vi "Main.vi"() -> ()   [LabVIEW 2021]
uses:
  <vilib>/myRIO/Common/Instrument Driver Framework/myRIO v1.0/Encoder/typedefs/Encoder Signal Mode.ctl
  <vilib>/Platform/TimedLoop/XDataNode/timing_clust.ctl
  <vilib>/Platform/TimedLoop/XDataNode/nitl_modes.ctl
  <vilib>/Platform/TimedLoop/XDataNode/wakeup.ctl
  <vilib>/myRIO/Common/Instrument Driver Framework/myRIO v1.0/UART/vis/myRIO v1.0 Close UART.vi
  <vilib>/Utility/error.llb/Error Cluster From Error Code.vi
  <vilib>/myRIO/Common/Instrument Driver Framework/myRIO v1.0/Encoder/vis/myRIO v1.0 Read Encoder.vi
  <vilib>/myRIO/Common/Instrument Driver Framework/myRIO v1.0/DIO/vis/myRIO v1.0 Read DIO.vi
  <vilib>/myRIO/Common/Instrument Driver Framework/myRIO v1.0/PWM/vis/myRIO v1.0 Write PWM.vi
  <vilib>/myRIO/Common/Instrument Driver Framework/Utilities/vis/FPGA Ref Manager.vi
  <vilib>/myRIO/Common/Instrument Driver Framework/myRIO v1.0/myRIO v1.0 Reset FPGA.vi
  <vilib>/myRIO/Common/Instrument Driver Framework/myRIO v1.0/IRQ/vis/myRIO v1.0 IRQ Info FGV.vi
  <vilib>/myRIO/Common/Instrument Driver Framework/myRIO v1.0/IRQ/vis/myRIO v1.0 Timer IRQ Info FGV.vi
  <vilib>/myRIO/Common/Instrument Driver Framework/myRIO v1.0/IRQ/vis/myRIO v1.0 ISR Agent.vi
  <vilib>/myRIO/Instrument Drivers/Utilities/vis/Reset Index.vi
  <vilib>/myRIO/Common/Instrument Driver Framework/myRIO v1.0/Resource Manager/vis/myRIO v1.0 Block Write Resource Manager.vi
  <vilib>/Platform/TimedLoop/XDataNode/XDataNode.xnode
  <vilib>/myRIO/Instrument Drivers/Onboard IO/Encoder/Encoder.lvlib
  <vilib>/myRIO/Instrument Drivers/Onboard IO/PWM/PWM.lvlib
  <vilib>/myRIO/Instrument Drivers/Utilities/Utilities.lvlib
  <vilib>/Platform/TimedLoop/XDataNode/XDNodeRunTimeDep.lvlib
  <vilib>/myRIO/Instrument Drivers/Onboard IO/DIO/DIO.lvlib
panel:
  in  "Limit Switch":bool
  out "Saved Measurement":dbl
  in  "stop":bool
  in  "Measure":bool
  in  "X":dbl(slide) scale=0.0..50.0
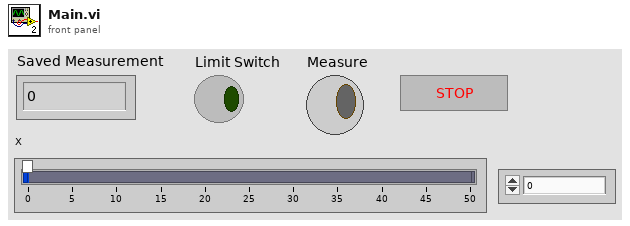
[diagram p1: front panel]
types:
  T1 = typedef "XDNodeRunTimeDep.lvlib/timing_clust.ctl" = cluster{"Expected End [f-1]":u64, "Actual End [f-1]":u64, "Finished Late? [f-1]":bool, "Expected End [i-1]":u64, "Actual End [i-1]":u64, "Finished Late? [i-1]":bool, "Expected Start [i]":u64, "Actual Start [i]":u64, "Expected Start [f]":u64, "Actual Start [f]":u64, "Source Name":string, "Structure Name":string, "Period":i64, "Deadline":i64, "Offset":i64, "Start":i64, "Priority":i32, "Timeout":i32, "Mode":T2, "Wakeup Reason":T3, "Error":errorcluster, "Source Type":string, "Secondary Source Type":string, "Global End Time":u64, "Global Start Time":u64, "Frame Duration":u64, "Iteration Duration":u64, "Assigned CPU":i32, "I/O Scan Engine Mode":u32}
  T2 = typedef "XDNodeRunTimeDep.lvlib/nitl_modes.ctl" = enum32{"No Change", "Process missed periods, maintain original phase", "Discard missed periods, maintain original phase", "Process missed periods, ignore original phase", "Discard missed periods, ignore original phase"}
  T3 = typedef "XDNodeRunTimeDep.lvlib/wakeup.ctl" = enum32{"Normal", "Aborted", "Asynchronous wakeup", "Timing source error", "Timed loop error", "Timeout"}
  T4 = enum8{"Enabled", "Disabled", "Disabled and Grayed Out"}
  T5 = typedef "Encoder Signal Mode.ctl" = enum16{"Quadrature phase signal", "Step and direction signal"}
  T6 = typedef "PWM.lvlib/PWM Reference.ctl" = cluster{"myRIO Reference":T7, "PWM Channels Enum":T11, "PWM Configuration":T12}
  T7 = typedef "myRIO Generic Hardware Reference.ctl" = cluster{"myRIO Model":T8, "myRIO Hardware Reference":T9}
  T8 = typedef "Hardware Version Enum.ctl" = enum16{"Unknown", "myRIO-1900", "myRIO-1950", "roboRIO", "NI ELVIS RIO CM", "ELVIS III"}
  T9 = typedef "myRIO v1.0 Reference.ctl" = cluster{"Generic FPGA Reference":T10, "Allow multiple opens":bool}
  T10 = typedef "Generic FPGA Reference.ctl" = refnum<k20>
  T11 = typedef "PWM Channels Enum.ctl" = enum16{"Not Connected", "C/PWM0", "C/PWM1", "A/PWM0", "A/PWM1", "A/PWM2", "A/PWM3", "A/PWM4", "A/PWM5", "A/PWM6", "A/PWM7", "A/PWM8", "A/PWM9", "A/PWM10", "A/PWM11", "A/PWM12", "A/PWM13", "A/PWM14", "A/PWM15", "A/PWM16", "A/PWM17", "A/PWM18", "A/PWM19", "B/PWM0", "B/PWM1", "B/PWM2", "B/PWM3", "B/PWM4", "B/PWM5", "B/PWM6", "B/PWM7", "B/PWM8", "B/PWM9", "B/PWM10", "B/PWM11", "B/PWM12", "B/PWM13", "B/PWM14", "B/PWM15", "B/PWM16", "B/PWM17", "B/PWM18", "B/PWM19", "PWM/PWM0", "PWM/PWM1", "PWM/PWM2", "PWM/PWM3", "PWM/PWM4", "PWM/PWM5", "PWM/PWM6", "PWM/PWM7", "PWM/PWM8", "PWM/PWM9"}
  T12 = typedef "PWM.lvlib/PWM Configuration.ctl" = cluster{"Frequency":dbl, "Duty Cycle":dbl}
  T13 = typedef "Encoder.lvlib/Encoder Reference.ctl" = cluster{"myRIO Reference":T7, "Encoder Channels Enum":T14}
  T14 = typedef "Encoder Channels Enum.ctl" = enum16{"Not Connected", "C/ENC0", "C/ENC1", "A/ENC", "A/ENC0", "A/ENC1", "A/ENC2", "A/ENC3", "A/ENC4", "A/ENC5", "A/ENC6", "A/ENC7", "A/ENC8", "A/ENC9", "B/ENC", "B/ENC0", "B/ENC1", "B/ENC2", "B/ENC3", "B/ENC4", "B/ENC5", "B/ENC6", "B/ENC7", "B/ENC8", "B/ENC9", "DIO/ENC0", "DIO/ENC1", "DIO/ENC2", "DIO/ENC3", "DIO/ENC4"}
  T15 = typedef "DIO.lvlib/DIO Reference.ctl" = cluster{"myRIO Reference":T7, "DIO Channels List":T16}
  T16 = typedef "DIO Channels List.ctl" = T17[]
  T17 = typedef "DIO Channels Enum.ctl" = enum16{"Not Connected", "C/DIO0", "C/DIO1", "C/DIO2", "C/DIO3", "C/DIO4", "C/DIO5", "C/DIO6", "C/DIO7", "A/DIO0", "A/DIO1", "A/DIO2", "A/DIO3", "A/DIO4", "A/DIO5", "A/DIO6", "A/DIO7", "A/DIO8", "A/DIO9", "A/DIO10", "A/DIO11", "A/DIO12", "A/DIO13", "A/DIO14", "A/DIO15", "A/DIO16", "A/DIO17", "A/DIO18", "A/DIO19", "B/DIO0", "B/DIO1", "B/DIO2", "B/DIO3", "B/DIO4", "B/DIO5", "B/DIO6", "B/DIO7", "B/DIO8", "B/DIO9", "B/DIO10", "B/DIO11", "B/DIO12", "B/DIO13", "B/DIO14", "B/DIO15", "B/DIO16", "B/DIO17", "B/DIO18", "B/DIO19", "LED0", "LED1", "LED2", "LED3", "Button0", "DIO/DIO0", "DIO/DIO1", "DIO/DIO2", "DIO/DIO3", "DIO/DIO4", "DIO/DIO5", "DIO/DIO6", "DIO/DIO7", "DIO/DIO8", "DIO/DIO9", "SPI/CS0", "SPI/CS1", "SPI/CS2", "SPI/CS3", "LED RADIO (Green)", "LED RADIO (Red)", "LED COMM (Green)", "LED COMM (Red)", "LED MODE (Green)", "LED MODE (Red)"}
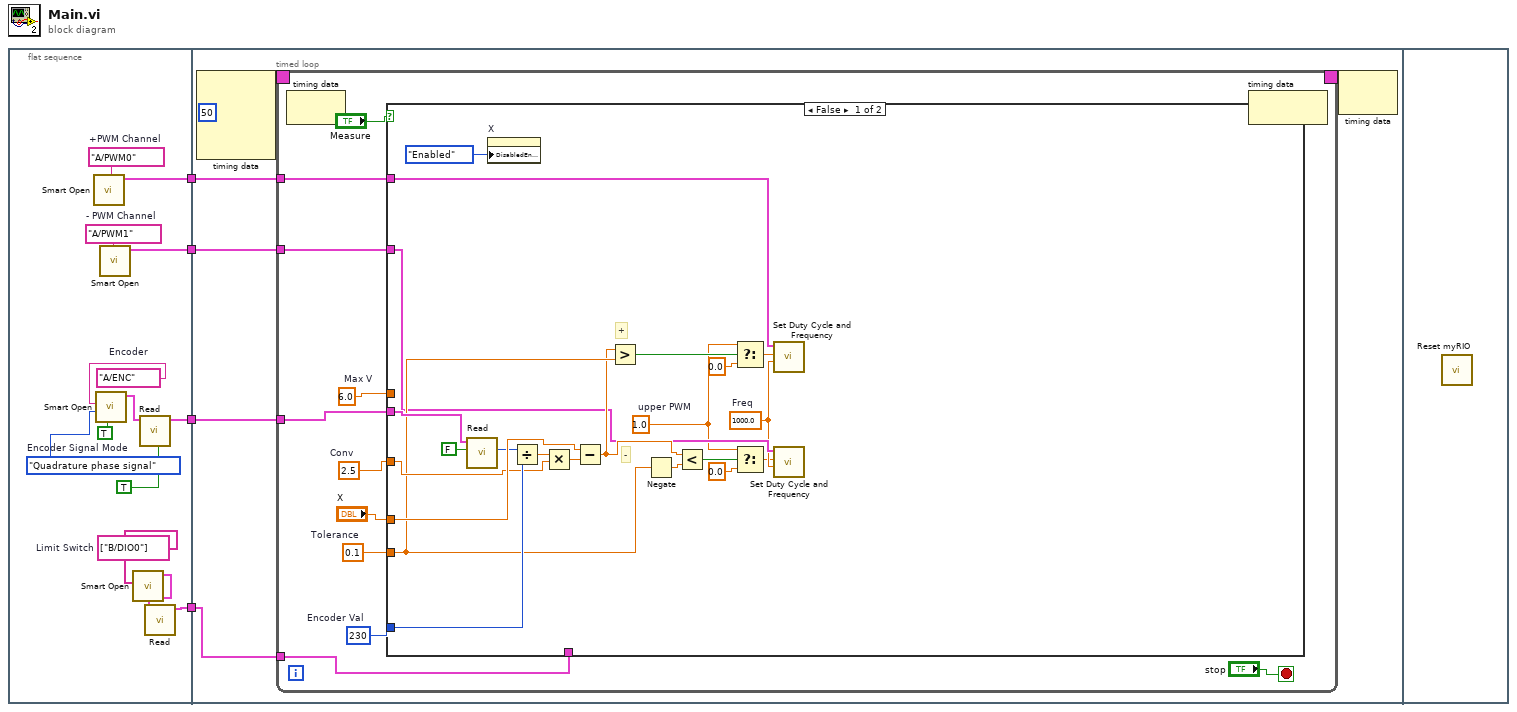
[diagram p0: block diagram]
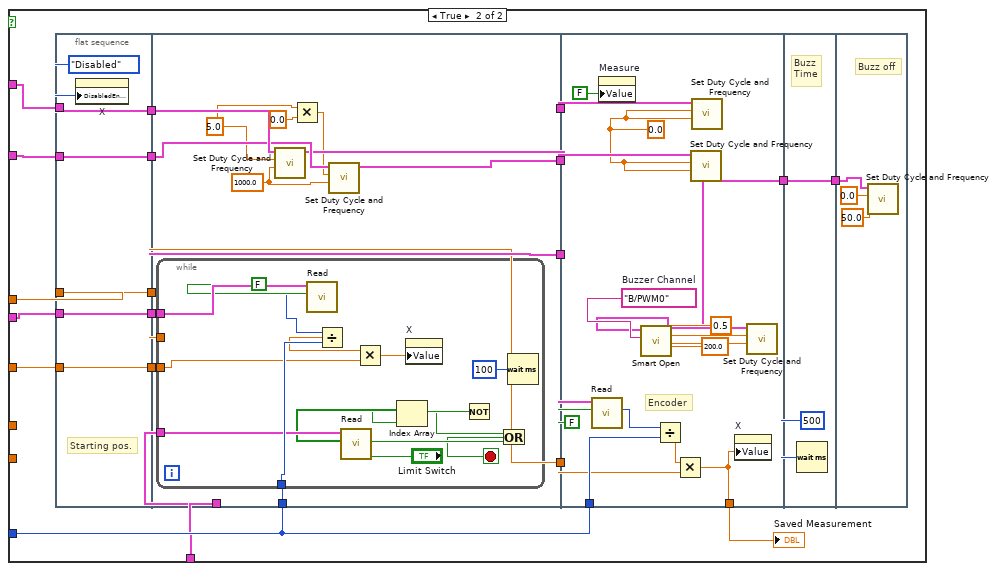
[diagram p2: hidden frame]
diagram:
  n1 = flat-sequence {
    tunnel: [w13] -> w4
    tunnel: [w10] -> w3
    tunnel: [w7] -> w2
    tunnel: [w6] -> w1
    tunnel: w4 -> [w21]
    tunnel: w3 -> [w20]
    tunnel: w2 -> [w19]
    tunnel: w1 -> [w18]
    frame #0 {
      w8 = tag "A/PWM1"  # - PWM Channel
      w9 = tag "A/PWM0"  # +PWM Channel
      w12 = tag[] ["B/DIO0"]  # Limit Switch
      w17 = Encoder_Signal_Mode."Quadrature phase signal"  # Encoder Signal Mode
      w5 = tag "A/ENC"  # Encoder
      n2 = call <vilib>:"Smart Open.vi"("Channel Name"=w9) -> ("PWM Ref Out"=w7:T6)  [unwired: 9 in, 1 out]
      n3 = call <vilib>:"Smart Open.vi"("Start Counter"=TRUE, "Encoder Signal Mode"=w17, "Channel Name"=w5) -> ("Encoder Ref Out"=w14:T13)  [unwired: 7 in, 1 out]
      n4 = call <vilib>:"Smart Open.vi"("Channel Name"=w8) -> ("PWM Ref Out"=w6:T6)  [unwired: 9 in, 1 out]
      n5 = call <vilib>:"Smart Open.vi"("Channel Names"=w12) -> ("DIO Ref Out"=w11:T15)  [unwired: 9 in, 1 out]
      n6 = call <vilib>:"Read.vi"("Reset Counter"=TRUE, "Encoder Ref In"=w14) -> ("Encoder Ref Out"=w13:T13)  [unwired: 5 in, 4 out]
      n7 = call <vilib>:"Read.vi"("DIO Ref In"=w11) -> ("DIO Ref Out"=w10:T15)  [unwired: 8 in, 2 out]
    }
    frame #1 {
      n8 = node-c288(i64 50 ("Period")) -> (w24:T1)  [unwired: 3 in]
      n9 = timed-loop {
        timing: w24 -> [_]
        timing-out: [_] -> w23
        tunnel: w21 -> [w30]
        tunnel: w20 -> [w29]
        tunnel: w19 -> [w28]
        tunnel: w18 -> [w27]
        stop <- "stop" stop-if-true
        w25 = 0.1  # Tolerance
        w26 = 2.5  # Conv
        w31 = 230  # Encoder Val
        w32 = 6.0  # Max V
        n10 = node-c288() -> ()  [unwired: 1 in, 1 out]
        n11 = case shown="False" "Measure" {
          tunnel: "X" -> [w57 _]
          tunnel: w32 -> [_ w78]
          tunnel: w31 -> [w58 w76]
          tunnel: w30 -> [w56 w72]
          tunnel: w29 -> [_ w71]
          tunnel: w28 -> [w45 w69]
          tunnel: w27 -> [w44 w67]
          tunnel: w26 -> [w51 w62]
          tunnel: w25 -> [w49 _]
          frame False {
            w40 = 1.0  # upper PWM
            w42 = 1000.0  # Freq
            # "-"
            # "+"
            n12 = call <vilib>:"Read.vi"("Reset Counter"=FALSE, "Encoder Ref In"=w56) -> ("Counter Value"=w54:i32)  [unwired: 5 in, 4 out]
            n13 = property on="X" class="Slide (strict)"("DisabledEnum"=T4."Enabled" ("Disabled")) -> ()  [unwired: 2 in, 2 out]
            n14 = Divide(x=w54, y=w58) -> (x/y=w53:dbl)
            n15 = Multiply(x=w53, y=w51) -> (x*y=w52:dbl)
            n16 = Subtract(x=w57, y=w52) -> (x-y=w48:dbl)
            n17 = Greater?(x=w48, y=w49) -> (0:w50:bool)
            n18 = Negate(x=w49) -> (-x=w41:dbl)
            n19 = Less?(x=w48, y=w41) -> (x < y?=w47:bool)
            n20 = Select(t=w40, s=w50, f=0.0 ("t")) -> (s? t:f=w38:dbl)
            n21 = Select(t=w40, s=w47, f=0.0) -> (s? t:f=w39:dbl)
            n22 = call <vilib>:"Set Duty Cycle and Frequency.vi"("Frequency [Hz]"=w42, "Duty Cycle"=w38, "PWM Ref In"=w45) -> ()  [unwired: 6 in, 2 out]
            n23 = call <vilib>:"Set Duty Cycle and Frequency.vi"("Frequency [Hz]"=w42, "Duty Cycle"=w39, "PWM Ref In"=w44) -> ()  [unwired: 6 in, 2 out]
          }
          frame True {
            n24 = flat-sequence {
              tunnel: w78 -> [w84]
              tunnel: [w84] -> w77
              tunnel: [w82] -> w73
              tunnel: w72 -> [w82]
              tunnel: w69 -> [w81]
              tunnel: [w81] -> w68
              tunnel: w67 -> [w80]
              tunnel: [w80] -> w66
              tunnel: w62 -> [w79]
              tunnel: [w79] -> w61
              tunnel: w77 -> [w97]
              tunnel: w76 -> [w96]
              tunnel: w73 -> [w94]
              tunnel: w71 -> [w95]
              tunnel: [w94] -> w70
              tunnel: w68 -> [w93]
              tunnel: w66 -> [w92]
              tunnel: [w89] -> w65
              tunnel: [w88] -> w64
              tunnel: w61 -> [w86]
              tunnel: [w86] -> w60
              tunnel: w76 -> [w126]
              tunnel: [w121] -> w75
              tunnel: w70 -> [w120]
              tunnel: w65 -> [w117]
              tunnel: w64 -> [w116]
              tunnel: [w113] -> w63
              tunnel: w60 -> [w112]
              tunnel: w75 -> [w128]
              tunnel: [w128] -> w74
              tunnel: w74 -> [w130]
              frame #0 {
                # "Starting pos."
                n25 = property on="X" class="Slide (strict)"("DisabledEnum"=T4."Disabled" ("Disabled")) -> ()  [unwired: 2 in, 2 out]
              }
              frame #1 {
                w90 = 1000.0 ("Frequency [Hz]")
                w85 = 5.0 ("Duty Cycle")
                n26 = while {
                  tunnel: w97 -> [_]
                  tunnel: w96 -> [w110]
                  tunnel: w94 -> [w108]
                  tunnel: w95 -> [w105]
                  tunnel: w86 -> [w99]
                  stop <- w103 stop-if-true
                  n27 = call <vilib>:"Read.vi"("Reset Counter"=FALSE, "Encoder Ref In"=w108) -> ("Counter Value"=w106:i32)  [unwired: 5 in, 4 out]
                  n28 = Divide(x=w106, y=w110) -> (x/y=w100:dbl)
                  n29 = call <vilib>:"Read.vi"("DIO Ref In"=w105) -> ("Values"=w104:bool[])  [unwired: 8 in, 2 out]
                  n30 = Multiply(x=w100, y=w99) -> (x*y=w98:dbl)
                  n31 = Index Array(array=w104) -> (element=w102:bool)  [unwired: 1 in]
                  n32 = property on="X" class="Slide (strict)"("Value"=w98) -> ()  [unwired: 2 in, 2 out]
                  n33 = Not(x=w102) -> (.not. x?=w101:bool)
                  n34 = Or(x=w101, y="Limit Switch") -> (x .or. y?=w103:bool)
                  n35 = Wait (ms)(milliseconds to wait=u32 100) -> ()  [unwired: 1 out]
                }
                n36 = call <vilib>:"Set Duty Cycle and Frequency.vi"("Frequency [Hz]"=w90, "Duty Cycle"=w85, "PWM Ref In"=w93) -> ("PWM Ref Out"=w89:T6)  [unwired: 6 in, 1 out]
                n37 = Multiply(x=w85, y=0.0) -> (x*y=w87:dbl)
                n38 = call <vilib>:"Set Duty Cycle and Frequency.vi"("Frequency [Hz]"=w90, "Duty Cycle"=w87, "PWM Ref In"=w92) -> ("PWM Ref Out"=w88:T6)  [unwired: 6 in, 1 out]
              }
              frame #2 {
                w125 = tag "B/PWM0"  # Buzzer Channel
                w115 = 0.0 ("Step size (Duty)")
                # "Encoder"
                n39 = call <vilib>:"Read.vi"("Reset Counter"=FALSE, "Encoder Ref In"=w120) -> ("Counter Value"=w118:i32)  [unwired: 5 in, 4 out]
                n40 = property on="Measure" class="Bool (strict)"("Value"=FALSE ("State control")) -> ()  [unwired: 2 in, 2 out]
                n41 = call <vilib>:"Smart Open.vi"("Channel Name"=w125) -> ("PWM Ref Out"=w124:T6)  [unwired: 9 in, 1 out]
                n42 = Divide(x=w118, y=w126) -> (x/y=w114:dbl)
                n43 = Multiply(x=w114, y=w112) -> (x*y=w113:dbl)
                n44 = call <vilib>:"Set Duty Cycle and Frequency.vi"("Frequency [Hz]"=w115, "Duty Cycle"=w115, "PWM Ref In"=w116) -> ()  [unwired: 6 in, 2 out]
                n45 = call <vilib>:"Set Duty Cycle and Frequency.vi"("Frequency [Hz]"=w115, "Duty Cycle"=w115, "PWM Ref In"=w117) -> ()  [unwired: 6 in, 2 out]
                n46 = property on="X" class="Slide (strict)"("Value"=w113) -> ()  [unwired: 2 in, 2 out]
                n47 = call <vilib>:"Set Duty Cycle and Frequency.vi"("Frequency [Hz]"=200.0, "Duty Cycle"=0.5, "PWM Ref In"=w124) -> ("PWM Ref Out"=w121:T6)  [unwired: 6 in, 1 out]
              }
              frame #3 {
                # "Buzz\nTime"
                n48 = Wait (ms)(milliseconds to wait=u32 500) -> ()  [unwired: 1 out]
              }
              frame #4 {
                # "Buzz off"
                n49 = call <vilib>:"Set Duty Cycle and Frequency.vi"("Frequency [Hz]"=50.0 ("Freq [Hz]"), "Duty Cycle"=0.0, "PWM Ref In"=w130) -> ()  [unwired: 6 in, 2 out]
              }
            }
            "Saved Measurement" <- w63
          }
        }
        n50 = node-c288() -> ()  [unwired: 1 in, 1 out]
      }
      n51 = node-c288(w23) -> ()  [unwired: 1 out]
    }
    frame #2 {
      n52 = call <vilib>:"Reset myRIO.vi"() -> ()  [unwired: 11 in, 1 out]
    }
  }
